vi "SVM Dense Train ONE_CLASS.vi"(7 "Options":T7={"cache_size"=200.0, "eps"=0.001, "shrinking"=TRUE, "probability"=FALSE}, 8 "error in (no error)":errorcluster, 9 "nu":T6=0.5 caption="nu (0,5)", 10 "Kernel":T8, 11 "Dense problem":T1) -> (0 "error out":errorcluster, 3 "Model":T2)   [LabVIEW 2014]
doc: "This function constructs and returns an SVM model according to the given training data and parameters."
uses:
  LibSVM Sparse/Controls/Kernel.ctl
  LibSVM Sparse/Wrapper API/Controls/svm_kernel_type.ctl
  LibSVM Sparse/Controls/Options Training.ctl
  LibSVM Sparse/Controls/Parameters ONE_CLASS.ctl
  Wrapper API/Controls/svmdense_model.ctl
  LibSVM Sparse/Wrapper API/Controls/svm_parameter.ctl
  LibSVM Sparse/Wrapper API/Controls/svm_type.ctl
  Wrapper API/Controls/svmdense_problem.ctl
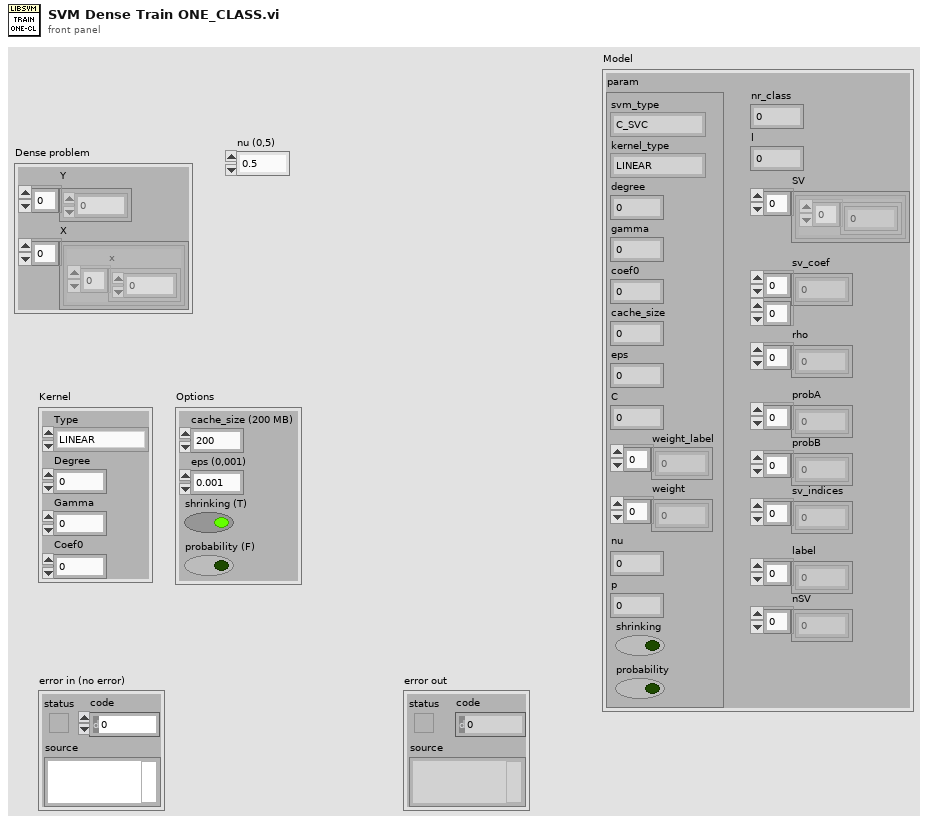
[diagram p1: front panel]
types:
  T1 = typedef "svmdense_problem.ctl" = cluster{"Y":dbl[], "X":cluster{"x":dbl[]}[]}
  T2 = typedef "svmdense_model.ctl" = cluster{"param":T3, "nr_class":i32, "l":i32, "SV":cluster{"Array":dbl[]}[], "sv_coef":dbl[][], "rho":dbl[], "probA":dbl[], "probB":dbl[], "sv_indices":i32[], "label":i32[], "nSV":i32[]}
  T3 = typedef "svm_parameter.ctl" = cluster{"svm_type":T4, "kernel_type":T5, "degree":i32, "gamma":dbl, "coef0":dbl, "cache_size":dbl, "eps":dbl, "C":dbl, "weight_label":i32[], "weight":dbl[], "nu":dbl, "p":dbl, "shrinking":bool, "probability":bool}
  T4 = typedef "svm_type.ctl" = enum32{"C_SVC", "NU_SVC", "ONE_CLASS", "EPSILON_SVR", "NU_SVR"}
  T5 = typedef "svm_kernel_type.ctl" = enum32{"LINEAR", "POLY", "RBF", "SIGMOID", "PRECOMPUTED"}
  T6 = typedef "Parameters ONE_CLASS.ctl" = dbl
  T7 = typedef "Options Training.ctl" = cluster{"cache_size":dbl, "eps":dbl, "shrinking":bool, "probability":bool}
  T8 = typedef "Kernel.ctl" = cluster{"Type":T5, "Degree":i32, "Gamma":dbl, "Coef0":dbl}
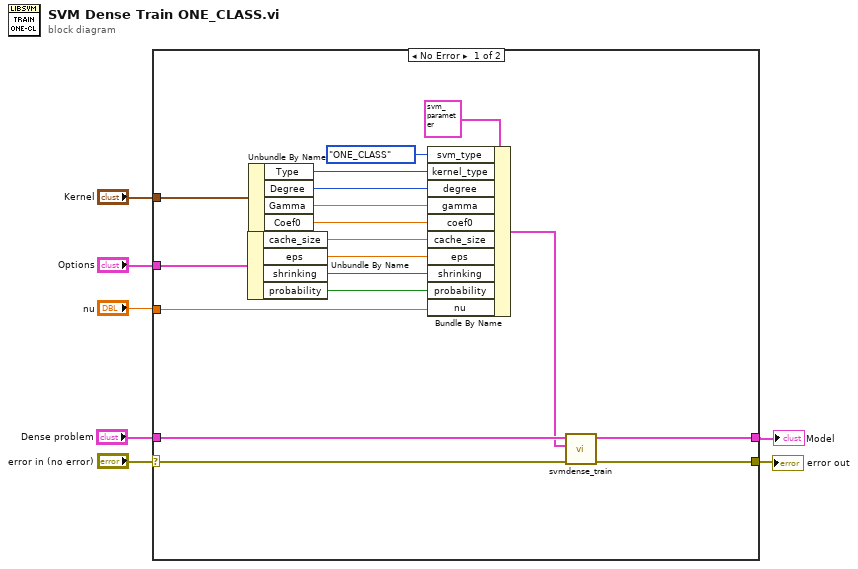
[diagram p0: block diagram]
diagram:
  n1 = case shown="No Error" "error in (no error)" {
    selector: "error in (no error)" -> [w8 w26]
    tunnel: [w9 w26] -> w7
    tunnel: "Dense problem" -> [w12 _]
    tunnel: "Kernel" -> [w24 _]
    tunnel: [w10 _] -> w1
    tunnel: "Options" -> [w16 _]
    tunnel: "nu" -> [w13 _]
    frame No Error {
      n2 = Unbundle By Name(w16) -> ("cache_size"=w18:dbl, "eps"=w17:dbl, "shrinking"=w15:bool, "probability"=w14:bool)
      n3 = Unbundle By Name(w24) -> ("Type"=w23:T5, "Degree"=w22:i32, "Gamma"=w21:dbl, "Coef0"=w20:dbl)
      n4 = Bundle By Name(cluster=T3 {"svm_type"=enum."C_SVC", "kernel_type"=enum."LINEAR", "degree"=0, "gamma"=0.0, "coef0"=0.0, "cache_size"=0.0, "eps"=0.0, "C"=0.0, "weight_label"=[], "weight"=[], "nu"=0.0, "p"=0.0, "shrinking"=FALSE, "probability"=FALSE} ("svm_parameter"), "svm_type"=svm_type."ONE_CLASS", "kernel_type"=w23, "degree"=w22, "gamma"=w21, "coef0"=w20, "cache_size"=w18, "eps"=w17, "shrinking"=w15, "probability"=w14, "nu"=w13) -> (w11:T3)
      n5 = call "svmdense_train.vi"("error in (no error)"=w8, "Parameters"=w11, "Problem"=w12) -> ("error out"=w9:errorcluster, "Model"=w10:T2)  [unwired: 7 in]
    }
    frame Error {
    }
  }
  "error out" <- w7
  "Model" <- w1
